vi "WS1050_AD7747_MeasCAP_Ver1.1.vi"(8 "error in (no error)":errorcluster, 9 "OFFSet Cal":dbl, 10 "AD7747_Number":string="8", 11 "Control":refnum<visa-resource-name>="COM8") -> (0 "error":errorcluster, 1 "CAP (pF)":string, 2 "CAP (pF)":dbl, 3 "Control out":refnum<visa-resource-name>, 4 "HEX":string)   [LabVIEW 2017]
uses:
  <vilib>/Utility/error.llb/whitespace.ctl
panel:
  # "Measure Cap Ad7747"
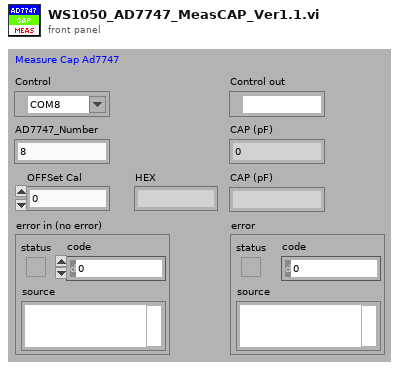
[diagram p1: front panel]
types:
  T1 = typedef "whitespace.ctl" = u16
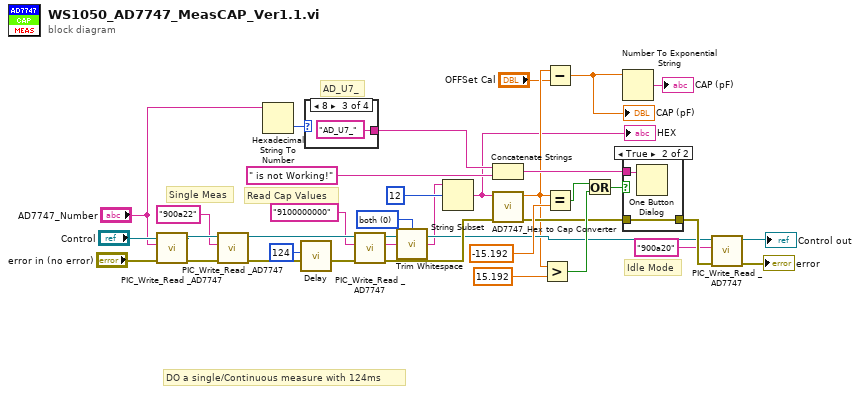
[diagram p0: block diagram]
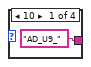
[diagram p2: hidden frame]
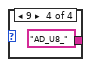
[diagram p4: hidden frame]
diagram:
  w1 = T1 0 items=["both", "start of string", "end of string"] ("location (both)")
  # "Single Meas"
  # "Idle Mode"
  # "Read Cap Values"
  # "DO a single/Continuous measure with 124ms"
  # "AD_U7_"
  n1 = call "PIC_Write_Read _AD7747.vi"("error in (no error)"="error in (no error)", "command"="AD7747_Number", "Control"="Control") -> ("error out"=w10:errorcluster, "Control out"=w34:refnum<visa-resource-name>)  [unwired: 6 in, 1 out]
  n2 = call "PIC_Write_Read _AD7747.vi"("error in (no error)"=w10, "command"="900a22" ("Data_In 2"), "Control"=w34) -> ("error out"=w6:errorcluster, "Control out"=w33:refnum<visa-resource-name>)  [unwired: 6 in, 1 out]
  n3 = Hexadecimal String To Number(string="AD7747_Number") -> (number=w20:u32)  [unwired: 2 in, 1 out]
  n4 = call "Delay.vi"("error in (no error)"=w6, "milliseconds to wait"=u32 124) -> ("error out"=w7:errorcluster)  [unwired: 9 in]
  n5 = case shown="8" w20 {
    tunnel: ["AD_U9_" _ "AD_U7_" "AD_U8_"] -> w23
    frame 10 {
    }
    frame 11, Default {
    }
    frame 8 {
    }
    frame 9 {
    }
  }
  n6 = call "PIC_Write_Read _AD7747.vi"("error in (no error)"=w7, "command"="9100000000" ("Data_In 2"), "Control"=w33) -> ("error out"=w36:errorcluster, "output"=w3:string, "Control out"=w17:refnum<visa-resource-name>)  [unwired: 6 in]
  n7 = call <vilib>:"Trim Whitespace.vi"("string"=w3, "location (both)"=w1) -> ("trimmed string"=w2:string)
  n8 = String Subset(string=w2, offset (0)=12) -> (substring=w4:string)  [unwired: 1 in]
  "HEX" <- w4
  n9 = Concatenate Strings(w23, " is not Working!" ("Offset Value 2")) -> (w21:string)
  n10 = call "AD7747_Hex to Cap Converter.vi"(8:w36, "HEX"=w4) -> (0:w28:errorcluster, "CAP (pF)"=w13:dbl)  [unwired: 7 in, 1 out]
  n11 = Greater?(x=w13, y=15.192) -> (0:w29:bool)
  n12 = Subtract(x=w13, y="OFFSet Cal") -> (x-y=w12:dbl)
  "CAP (pF)" <- w12
  n13 = Equal?(x=w13, y=-15.192) -> (x = y?=w30:bool)
  n14 = Or(x=w30, y=w29) -> (x .or. y?=w27:bool)
  n15 = Number To Exponential String(number=w12) -> (E-format string=→"CAP (pF)":string)  [unwired: 3 in]
  n16 = case shown="True" w27 {
    tunnel: w28 -> [w40 w42]
    tunnel: [w40 w42] -> w19
    tunnel: w21 -> [_ w41]
    frame False {
    }
    frame True {
      n17 = One Button Dialog(message=w41) -> ()  [unwired: 1 in, 1 out]
    }
  }
  n18 = call "PIC_Write_Read _AD7747.vi"("error in (no error)"=w19, "command"="900a20" ("Data_In 2"), "Control"=w17) -> ("error out"=→"error":errorcluster, "Control out"=→"Control out":refnum<visa-resource-name>)  [unwired: 6 in, 1 out]
